vi "Start Testing.vi"(8 "error in (no error)":errorcluster, 9 "Test Settings":T1 {"Lateral Load Cell Sensitivity" format="%.6f"; "Axial Load Cell Sensitivity" format="%.6f"}, 10 "Model in":refnum<class "Model.lvclass">, 11 "Wait For User Input State in":refnum<class "Wait For User Input State.lvclass">) -> (0 "error out":errorcluster, 2 "Model out":refnum<class "Model.lvclass">, 3 "Wait For User Input State out":refnum<class "Wait For User Input State.lvclass">)   [LabVIEW 2016, in "Wait For User Input State.lvclass"]
uses:
  Wait For User Input State.lvclass
  Model/Model/Model.lvclass
  Typedefs/TestSettings.ctl
  Common_RT_FAILC/DataTypes/FATypes.ctl
  Typedefs/StateTypes.ctl
  Common_RT_FAILC/FAILCFactory/FAILCFactory.lvclass
  Model/Model/Model.lvclass/Model.ctl
  Typedefs/FAMT Typedefs.lvlib
  Model/Boot Loader/Boot Loader.lvclass
  Common_RT_FAILC/RTFAILC.lvlib
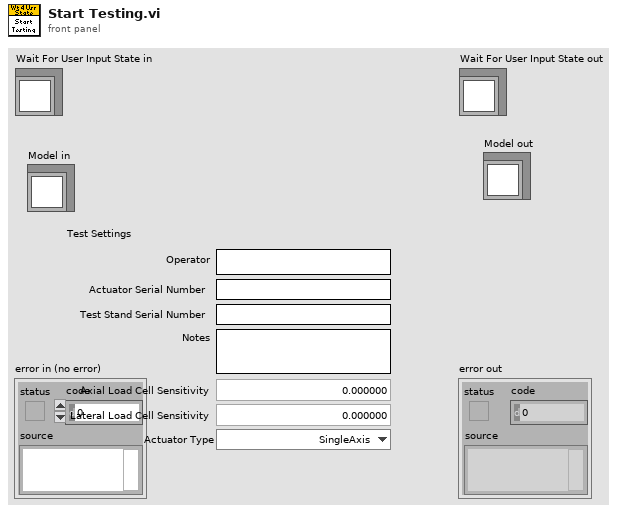
[diagram p1: front panel]
types:
  T1 = typedef "FAMT Typedefs.lvlib/TestSettings.ctl" = cluster{"Operator":string, "Notes":string, "Actuator Serial Number":string, "Test Stand Serial Number":string, "Axial Load Cell Sensitivity":dbl, "Lateral Load Cell Sensitivity":dbl, "Actuator Type":T2}
  T2 = typedef "RTFAILC.lvlib/FATypes.ctl" = enum16{"SingleAxis", "LateralDualAxis", "CrossLateralDualAxis"}
  T3 = typedef "FAMT Typedefs.lvlib/StateTypes.ctl" = enum16{"Offline State", "Fault State", "Standby State", "Disabled State", "Enabled State", "Wait For User Input State", "Test Actuator State"}
  T4 = typedef "RTFAILC.lvlib/FASettings.ctl" = cluster{"ILCSettings":T5, "ID":i16, "FATypes":T2}
  T5 = typedef "RTILC.lvlib/ILCSettings.ctl" = cluster{"Subnet":u8, "Address":u8}
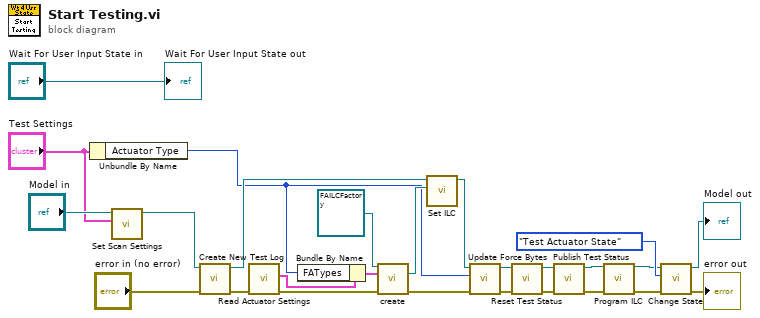
[diagram p0: block diagram]
diagram:
  n1 = Unbundle By Name("Test Settings") -> ("Actuator Type"=w10:T2)
  n2 = call "Set Scan Settings.vi"("Test Settings"="Test Settings", "Model in"="Model in") -> ("Model out"=w20:refnum<class "Model.lvclass">)  [unwired: 9 in]
  n3 = call "Create New Test Log.vi"("error in (no error)"="error in (no error)", "Model in"=w20) -> ("error out"=w15:errorcluster, "Model out"=w12:refnum<class "Model.lvclass">)  [unwired: 8 in]
  n4 = call "Read Actuator Settings.vi"("error in (no error)"=w15) -> ("error out"=w14:errorcluster, "FASettings"=w18:T4)  [unwired: 8 in, 1 out]
  n5 = Bundle By Name(cluster=w18, "FATypes"=w10) -> (w17:T4)
  n6 = call "create.vi"("FAILCFactory in"=refnum<class "FAILCFactory.lvclass"> refnum ("RTFAILC.lvlib:FAILCFactory.lvclass"), "FASettings"=w17, "error in (no error)"=w14) -> ("ForceActuator"=w13:refnum<class "FAILC.lvclass">, "error out"=w9:errorcluster)  [unwired: 10 in, 1 out]
  n7 = call "Set ILC.vi"("ILC"=w13, "Model in"=w12) -> ("Model out"=w11:refnum<class "Model.lvclass">)  [unwired: 9 in]
  n8 = call "Update Force Bytes.vi"("error in (no error)"=w9, "FATypes"=w10, "Model in"=w11) -> ("error out"=w6:errorcluster, "Model out"=w8:refnum<class "Model.lvclass">)  [unwired: 7 in]
  n9 = call "Reset Test Status.vi"("error in (no error)"=w6, "Model in"=w8) -> ("error out"=w5:errorcluster, "Model out"=w7:refnum<class "Model.lvclass">)  [unwired: 8 in]
  n10 = call "Publish Test Status.vi"("error in (no error)"=w5, "Model in"=w7) -> ("error out"=w3:errorcluster, "Model out"=w4:refnum<class "Model.lvclass">)  [unwired: 8 in]
  n11 = call "Program ILC.vi"("Model in"=w4, "error in (no error)"=w3) -> ("Model out"=w2:refnum<class "Model.lvclass">, "error out"=w1:errorcluster)  [unwired: 12 in]
  n12 = call "Change State.vi"("error in (no error)"=w1, "State Types"=StateTypes."Test Actuator State" ("State:"), "Model in"=w2) -> ("error out"=→"error out":errorcluster, "Model out"=→"Model out":refnum<class "Model.lvclass">)  [unwired: 7 in]
  "Wait For User Input State out" <- "Wait For User Input State in"
